vi "Display Load Menu Delete.vi"(8 "error in":errorcluster, 9 "Display Name":string, 10 "Node In":string, 11 "VISA resource name":refnum<visa-resource-name>) -> (0 "error out":errorcluster, 2 "Node Out":string, 3 "VISA resource name out":refnum<visa-resource-name>, 4 "Command String":string)   [LabVIEW 2018, in "Keithley 2600 Series.lvlib"]
doc: "This VI removes an entry from the \"USER TESTS\" submenu of the \"LOAD TEST\" menu.\n\n<b>Functions and Attributes Used</b>\ndisplay.loadmenu.delete()"
uses:
  Keithley 2600 Series.lvlib
  Private/GlobalVariables.vi
panel:
  # "(c) 2008 Keithley Instruments, Inc.  ALL RIGHTS RESERVED."
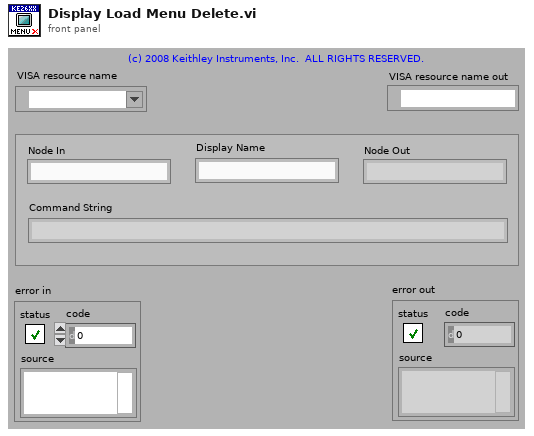
[diagram p1: front panel]
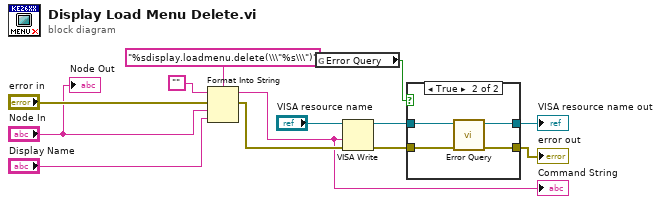
[diagram p0: block diagram]
diagram:
  n1 = Format Into String(format string="%sdisplay.loadmenu.delete(\\\"%s\\\")", initial string="", error in="error in", "Node In", "Display Name") -> (resulting string=w1:string, error out=w8:errorcluster)
  "Command String" <- w1
  n2 = global read "GlobalVariables.vi" "Error Query"() -> (w4:bool)
  n3 = VISA Write(VISA resource name="VISA resource name", write buffer=w1, error in (no error)=w8) -> (VISA resource name out=w6:refnum<visa-resource-name>, error out=w5:errorcluster)  [unwired: 1 out]
  n4 = case shown="True" w4 {
    tunnel: w6 -> [w15 w19]
    tunnel: w5 -> [w14 w18]
    tunnel: [w15 w17] -> w2
    tunnel: [w14 w16] -> w3
    frame False {
    }
    frame True {
      n5 = call "Error Query.vi"("error in (no error)"=w18, "VISA resource name"=w19) -> ("error out"=w16:errorcluster, "VISA resource name out"=w17:refnum<visa-resource-name>)  [unwired: 8 out]
    }
  }
  "VISA resource name out" <- w2
  "error out" <- w3
  "Node Out" <- "Node In"
